vi "While Loop.vi"() -> ()   [LabVIEW 2015, in "Simple Progress Bar.lvlib"]
uses:
  New Job Status.vi
  New Item Progression.vi
  Class/Finish.vi
  Simple Progress Bar.lvlib
  Class/Bar.lvclass
panel:
  out "error out":errorcluster
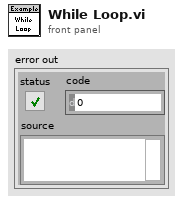
[diagram p1: front panel]
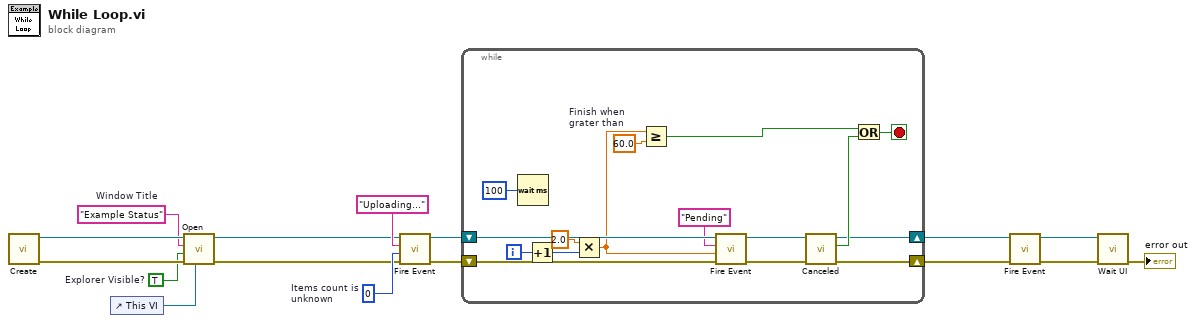
[diagram p0: block diagram]
diagram:
  w3 = 0  # Items count is  unknown
  w8 = "Example Status"  # Window Title
  w10 = TRUE  # Explorer Visible?
  n1 = call "Create.vi"() -> ("error out"=w12:errorcluster, "Bar out"=w9:refnum<class "Bar.lvclass">)  [unwired: 10 in]
  n2 = control-ref of="This VI"() -> (w11:refnum<vi>)
  n3 = call "Open.vi"("VI"=w11, "error in (no error)"=w12, "Explorer Visible? (F)"=w10, "Window Title"=w8, "Bar in"=w9) -> ("error out"=w1:errorcluster, "Bar out"=w2:refnum<class "Bar.lvclass">)  [unwired: 5 in]
  n4 = call-poly "Fire Event.vi"("error in (no error)"=w1, "Items (unknown)"=w3, "Status"="Uploading...", "Bar in"=w2) -> ("error out"=w5:errorcluster, "Bar out"=w6:refnum<class "Bar.lvclass">)  [unwired: 6 in]
  n5 = while {
    shift-right: [w22] -> w14
    shift-left: w5 -> [w28]
    shift-right: [w18] -> w13
    shift-left: w6 -> [w27]
    i -> [w30]
    stop <- w21 stop-if-true
    w24 = 60.0  # Finish when  grater than
    n6 = Wait (ms)(milliseconds to wait=u32 100) -> ()  [unwired: 1 out]
    n7 = Increment(x=w30) -> (x+1=w29:i32)
    n8 = Multiply(x=2.0, y=w29) -> (x*y=w25:dbl)
    n9 = Greater Or Equal?(x=w25, y=w24) -> (x >= y?=w23:bool)
    n10 = call-poly "Fire Event.vi"("error in (no error)"=w28, "Progression"=w25, "Status"="Pending", "Bar in"=w27) -> ("error out"=w17:errorcluster, "Bar out"=w19:refnum<class "Bar.lvclass">)  [unwired: 6 in]
    n11 = call "Canceled.vi"("error in (no error)"=w17, "Bar in"=w19) -> ("error out"=w22:errorcluster, "Canceled by user?"=w20:bool, "Bar out"=w18:refnum<class "Bar.lvclass">)  [unwired: 7 in]
    n12 = Or(x=w23, y=w20) -> (x .or. y?=w21:bool)
  }
  n13 = call-poly "Fire Event.vi"("error in (no error)"=w14, "Bar in"=w13) -> ("error out"=w15:errorcluster, "Bar out"=w7:refnum<class "Bar.lvclass">)  [unwired: 8 in]
  n14 = call "Wait UI.vi"("error in (no error)"=w15, "Bar in"=w7) -> ("error out"=→"error out":errorcluster)  [unwired: 6 in, 3 out]
